vi "移位寄存器（菲波那切数列）.vi"() -> ()   [LabVIEW 2017]
panel:
  out "数组":i32[](array[numeric])
  out "数值":u64
  out "x+y":u64
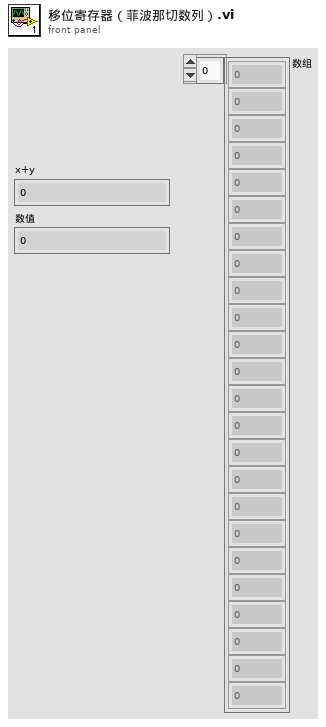
[diagram p1: front panel]
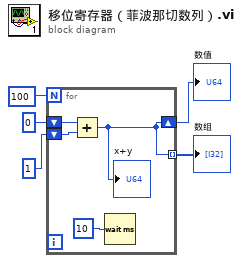
[diagram p0: block diagram]
diagram:
  n1 = for {
    N: 100 -> [_]
    shift-right: [w6] -> w3
    shift-left: 0 -> [w9]
    shift-left: 1 -> [w8]
    tunnel: [w6] -> w1 mode=indexing
    n2 = Add(x=w9, y=w8) -> (x+y=w6:i32)
    "x+y" <- w6
    n3 = Wait (ms)(milliseconds to wait=10) -> ()  [unwired: 1 out]
  }
  "数值" <- w3
  "数组" <- w1
